vi "PH_TKTDS-30xx.Evt Call Set Channel Configuration.vi"(0 "i ref in":refnum<vi>, 1 "Instance":string="N/A", 2 "GUI Element Name":string="N/A", 3 "Channel Configuration":T1={"Channel Name"="CH1", "Input Impedance"="MEG", "Max Input Frequency"="TWENTY", "Vertical Coupling"=1, "Channel Enabled"=TRUE, "Probe Attenuation"=1.0, "Vertical Range"=100.0, "Vertical Offset"=0.0} {"Vertical Offset" format="%#_6p"; "Vertical Range" items=["1mV"=0.001, "2mV"=0.002, "5mV"=0.005, "10mV"=0.01, "20mV"=0.02, "50mV"=0.05, "100mV"=0.1, "200mV"=0.2, "500mV"=0.5, "1V"=1.0]; "Probe Attenuation" format="%#.2f"}, 5 "error in (no error)":errorcluster) -> (14 "i ref out":refnum<vi>, 19 "error out":errorcluster)   [LabVIEW 2014, in "PH_TKTDS-30xx.lvlib"]
doc: "This VI calls sets a simple call."
uses:
  PH_TKTDS-30xx.lvlib
  PH_TKTDS-30xx.Channel Config.ctl
  CS_Core/CSSystem/CoreLib/CoreLib.double 2 byte array.vi
  CS_Core/CSSystem/CoreLib/CoreLib.short 2 byte array.vi
  CS_Core/CSSystem/CoreLib/CoreLib.int 2 byte array.vi
  CS_Core/CSSystem/CoreLib/CoreLib.string 2 byte array.vi
  CS_Core/CSSystem/CoreLib/CoreLib.lvlib
  CS_Core/BaseProcess/BaseProcess.lvlib
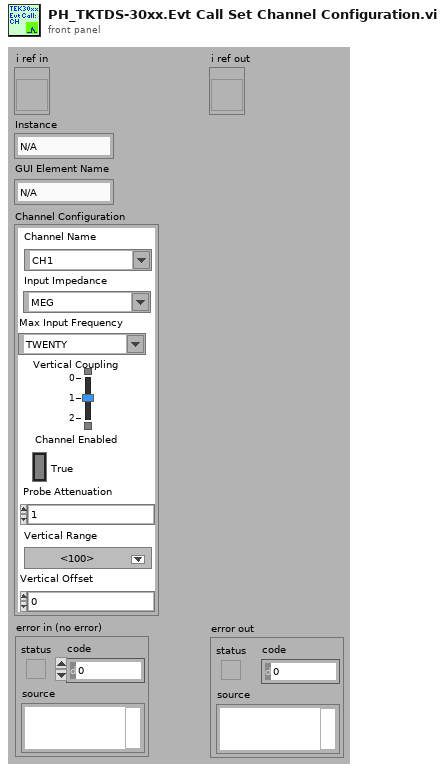
[diagram p1: front panel]
types:
  T1 = typedef "PH_TKTDS-30xx.lvlib/PH_TKTDS-30xx.Channel Config.ctl" = cluster{"Channel Name":string, "Input Impedance":string, "Max Input Frequency":string, "Vertical Coupling":i32, "Channel Enabled":bool, "Probe Attenuation":dbl, "Vertical Range":dbl, "Vertical Offset":dbl}
  T2 = typedef "CoreDefs.rawDataType.ctl" = i8[]
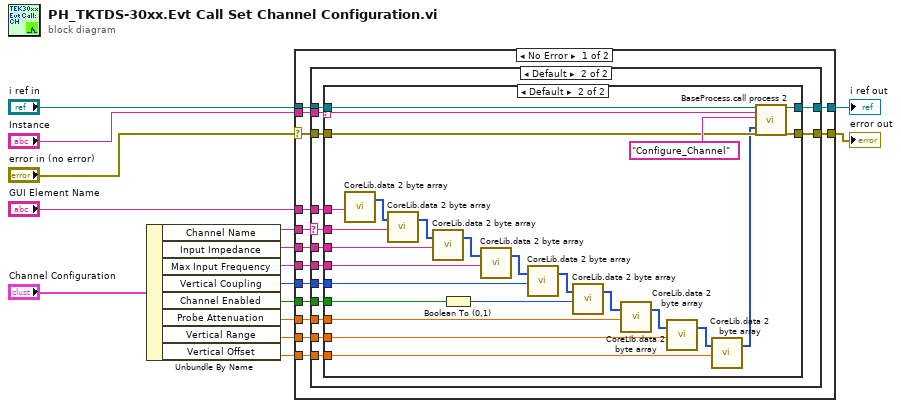
[diagram p0: block diagram]
diagram:
  n1 = Unbundle By Name("Channel Configuration") -> ("Channel Name"=w9:string, "Input Impedance"=w8:string, "Max Input Frequency"=w7:string, "Vertical Coupling"=w6:i32, "Channel Enabled"=w5:bool, "Probe Attenuation"=w4:dbl, "Vertical Range"=w3:dbl, "Vertical Offset"=w2:dbl)
  n2 = case shown="No Error" "error in (no error)" {
    selector: "error in (no error)" -> [w25 w73]
    tunnel: [w29 w74] -> w15
    tunnel: [w28 w73] -> w14
    tunnel: "i ref in" -> [w27 w74]
    tunnel: w9 -> [w24 _]
    tunnel: "Instance" -> [w26 _]
    tunnel: w8 -> [w23 _]
    tunnel: w7 -> [w22 _]
    tunnel: w6 -> [w21 _]
    tunnel: w5 -> [w20 _]
    tunnel: w4 -> [w19 _]
    tunnel: w3 -> [w18 _]
    tunnel: w2 -> [w17 _]
    tunnel: "GUI Element Name" -> [w16 _]
    frame No Error {
      n3 = case shown="Default" w24 {
        selector: w24 -> [_ w40]
        tunnel: [w31 w45] -> w29
        tunnel: [w30 w44] -> w28
        tunnel: w27 -> [w31 w43]
        tunnel: w26 -> [_ w42]
        tunnel: w25 -> [w30 w41]
        tunnel: w23 -> [_ w39]
        tunnel: w22 -> [_ w38]
        tunnel: w21 -> [_ w37]
        tunnel: w20 -> [_ w36]
        tunnel: w19 -> [_ w35]
        tunnel: w18 -> [_ w34]
        tunnel: w17 -> [_ w33]
        tunnel: w16 -> [_ w32]
        frame "", "N/A" {
        }
        frame Default {
          n4 = case shown="Default" w42 {
            selector: w42 -> [_ w67]
            tunnel: [w46 w71] -> w45
            tunnel: [w47 w70] -> w44
            tunnel: w43 -> [w46 w69]
            tunnel: w41 -> [w47 w68]
            tunnel: w40 -> [_ w66]
            tunnel: w39 -> [_ w65]
            tunnel: w38 -> [_ w63]
            tunnel: w37 -> [_ w58]
            tunnel: w36 -> [_ w57]
            tunnel: w35 -> [_ w55]
            tunnel: w34 -> [_ w52]
            tunnel: w33 -> [_ w51]
            tunnel: w32 -> [_ w48]
            frame "N/A" {
            }
            frame Default {
              n5 = call-poly "CoreLib.data 2 byte array.vi"("string"=w48) -> ("byteArray out"=w49:T2)  [unwired: 18 in]
              n6 = call-poly "CoreLib.data 2 byte array.vi"("byteArray"=w49, "string"=w66) -> ("byteArray out"=w64:T2)  [unwired: 17 in]
              n7 = call-poly "CoreLib.data 2 byte array.vi"("byteArray"=w64, "string"=w65) -> ("byteArray out"=w62:T2)  [unwired: 17 in]
              n8 = Boolean To (0,1)(Boolean=w57) -> (0, 1=w56:i16)
              n9 = call-poly "CoreLib.data 2 byte array.vi"("byteArray"=w62, "string"=w63) -> ("byteArray out"=w54:T2)  [unwired: 17 in]
              n10 = call-poly "CoreLib.data 2 byte array.vi"("byteArray"=w54, "i32"=w58) -> ("byteArray out"=w61:T2)  [unwired: 17 in]
              n11 = call-poly "CoreLib.data 2 byte array.vi"("byteArray"=w61, "i16"=w56) -> ("byteArray out"=w60:T2)  [unwired: 17 in]
              n12 = call-poly "CoreLib.data 2 byte array.vi"("byteArray"=w60, "f64"=w55) -> ("byteArray out"=w53:T2)  [unwired: 17 in]
              n13 = call-poly "CoreLib.data 2 byte array.vi"("byteArray"=w53, "f64"=w52) -> ("byteArray out"=w59:T2)  [unwired: 17 in]
              n14 = call-poly "CoreLib.data 2 byte array.vi"("byteArray"=w59, "f64"=w51) -> ("byteArray out"=w50:T2)  [unwired: 17 in]
              n15 = call "BaseProcess.call process 2.vi"("i ref in"=w69, "Object"=w67, "Selector"="Configure_Channel", "Data"=w50, "error in (no error)"=w68) -> ("i ref out"=w71:refnum<vi>, "error out"=w70:errorcluster)  [unwired: 13 in]
            }
          }
        }
      }
    }
    frame Error {
    }
  }
  "i ref out" <- w15
  "error out" <- w14
